vi "Assert Elements are Homogeneous.vi"(8 "error in (no error)":errorcluster, 11 "array in":variant[](array[variant])) -> (0 "error out":errorcluster, 3 "array out":variant[](array[variant]))   [LabVIEW 2017, in "Variant Data Manipulation.lvlib"]
uses:
  <vilib>/National Instruments/Variant Data Manipulation/Variant Data Manipulation.lvlib
  <vilib>/Utility/Data Type/NI_Data Type.lvlib
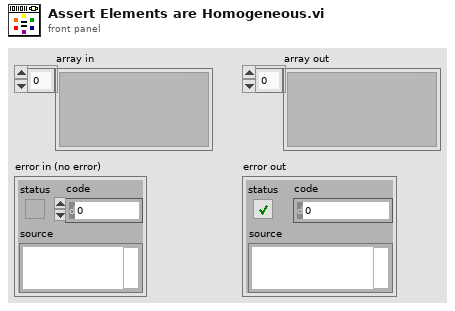
[diagram p1: front panel]
types:
  T1 = typedef "NI_Data Type.lvlib/Data Type.ctl" = enum8{"Invalid Type", "Void", "I8", "I16", "I32", "I64", "U8", "U16", "U32", "U64", "Single Float", "Double Float", "Extended Float", "Single Complex", "Double Complex", "Extended Complex", "Enum U8", "Enum U16", "Enum U32", "Enum U64", "Single Float With Unit", "Double Float With Unit", "Extended Float With Unit", "Single Complex with Unit", "Double Complex with Unit", "Extended Complex with Unit", "Boolean", "String", "Path", "Picture", "Tag", "Array", "Cluster", "Variant", "LV Variant", "Waveform", "Timestamp", "Digital Waveform", "Digital Data", "ExpressData", "Refnum", "External Data", "VI", "Poly VI", "LabVIEW Class Instance", "Fixed Point"}
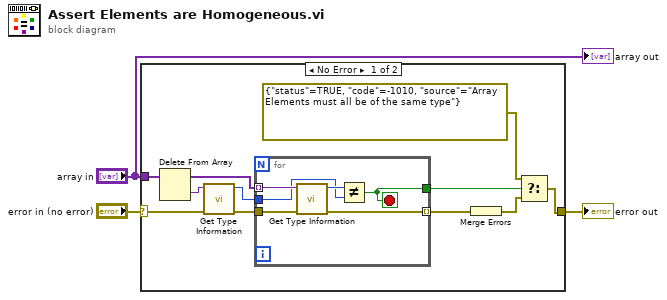
[diagram p0: block diagram]
diagram:
  n1 = case shown="No Error" "error in (no error)" {
    selector: "error in (no error)" -> [w10 w21]
    tunnel: "array in" -> [w11 _]
    tunnel: [w4 w21] -> w1
    frame No Error {
      n2 = Delete From Array(array=w11) -> (deleted portion=w13:variant, array with subset deleted=w12:variant[])  [unwired: 2 in]
      n3 = call <vilib>:"Get Type Information.vi"("error in (no error)"=w10, "Variant"=w13) -> ("error out"=w9:errorcluster, "Type"=w14:T1)  [unwired: 5 in, 3 out]
      n4 = for {
        tunnel: w12 -> [w20] mode=indexing
        tunnel: w14 -> [w18]
        tunnel: [w17] -> w7
        tunnel: w9 -> [w16]
        tunnel: [w15] -> w8 mode=indexing
        stop <- w17 stop-if-true
        n5 = call <vilib>:"Get Type Information.vi"("error in (no error)"=w16, "Variant"=w20) -> ("error out"=w15:errorcluster, "Type"=w19:T1)  [unwired: 5 in, 3 out]
        n6 = Not Equal?(x=w19, y=w18) -> (x != y?=w17:bool)
      }
      n7 = Merge Errors(w8) -> (w6:errorcluster)
      n8 = Select(t=errorcluster {"status"=TRUE, "code"=-1010, "source"="Array Elements must all be of the same type"}, s=w7, f=w6) -> (s? t:f=w4:errorcluster)
    }
    frame Error {
    }
  }
  "error out" <- w1
  "array out" <- "array in"
